vi "teste carga suporte.vi"() -> ()   [LabVIEW 2020]
panel:
  in  "Flecha alvo":dbl=12.266613074311236 format="%#_13g"
  out "Fs":dbl
  in  "As":dbl
  out "T0s":dbl
  in  "ps":dbl
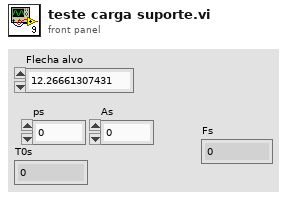
[diagram p1: front panel]
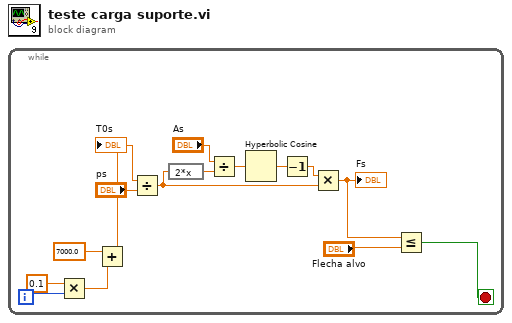
[diagram p0: block diagram]
diagram:
  n1 = while {
    i -> [w5]
    stop <- w6 stop-if-true
    n2 = Multiply(x=0.1, y=w5) -> (x*y=w3:dbl)
    n3 = Add(x=7000.0, y=w3) -> (x+y=w2:dbl)
    "T0s" <- w2
    n4 = Divide(x=w2, y="ps") -> (x/y=w14:dbl)
    n5 = expression code="2*x"(w14) -> (w13:dbl)
    n6 = Divide(x="As", y=w13) -> (x/y=w11:dbl)
    n7 = Hyperbolic Cosine(1:w11) -> (0:w10:dbl)
    n8 = Decrement(x=w10) -> (x-1=w15:dbl)
    n9 = Multiply(x=w15, y=w14) -> (x*y=w8:dbl)
    "Fs" <- w8
    n10 = Less Or Equal?(x=w8, y="Flecha alvo") -> (x <= y?=w6:bool)
  }
